vi "Agilis-Commands.vi"(6 "raw in":string="1ve?\r\n", 7 "Command in":T1(ring), 8 "error in (no error)":errorcluster, 9 "Value":dbl, 10 "Axis in":u8=1, 11 "VISA Refnum in":refnum<visa-resource-name>) -> (0 "error out":errorcluster, 1 "value":dbl format="%#.6g", 3 "VISA resource name out":refnum<visa-resource-name>, 4 "read buffer":string)   [LabVIEW 2011]
uses:
  <vilib>/Instr/_visa.llb/VISA Flush IO Buffer Mask.ctl
panel:
  out "sent":string
  out "return count":u32
  # "Staus x28: moving\nstatus x33_d51: OK\nstatus 10: no init?\nError 64:OK\nError:72 no init"
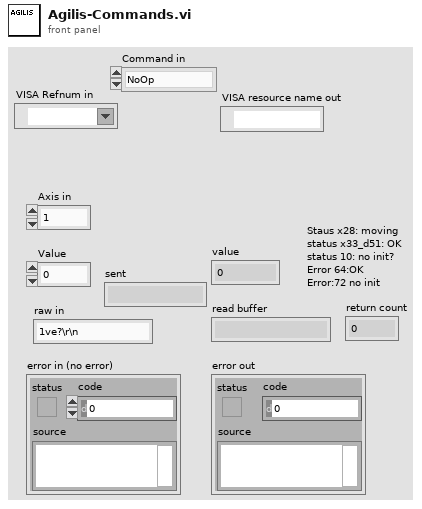
[diagram p1: front panel]
types:
  T1 = enum16{"NoOp", "GetStatus", "GetPosition", "SetPosition", "SetRelative", "GetError", "WriteRawAndRead", "clear", "switchOn"}
  T2 = typedef "VISA Flush IO Buffer Mask.ctl" = u16
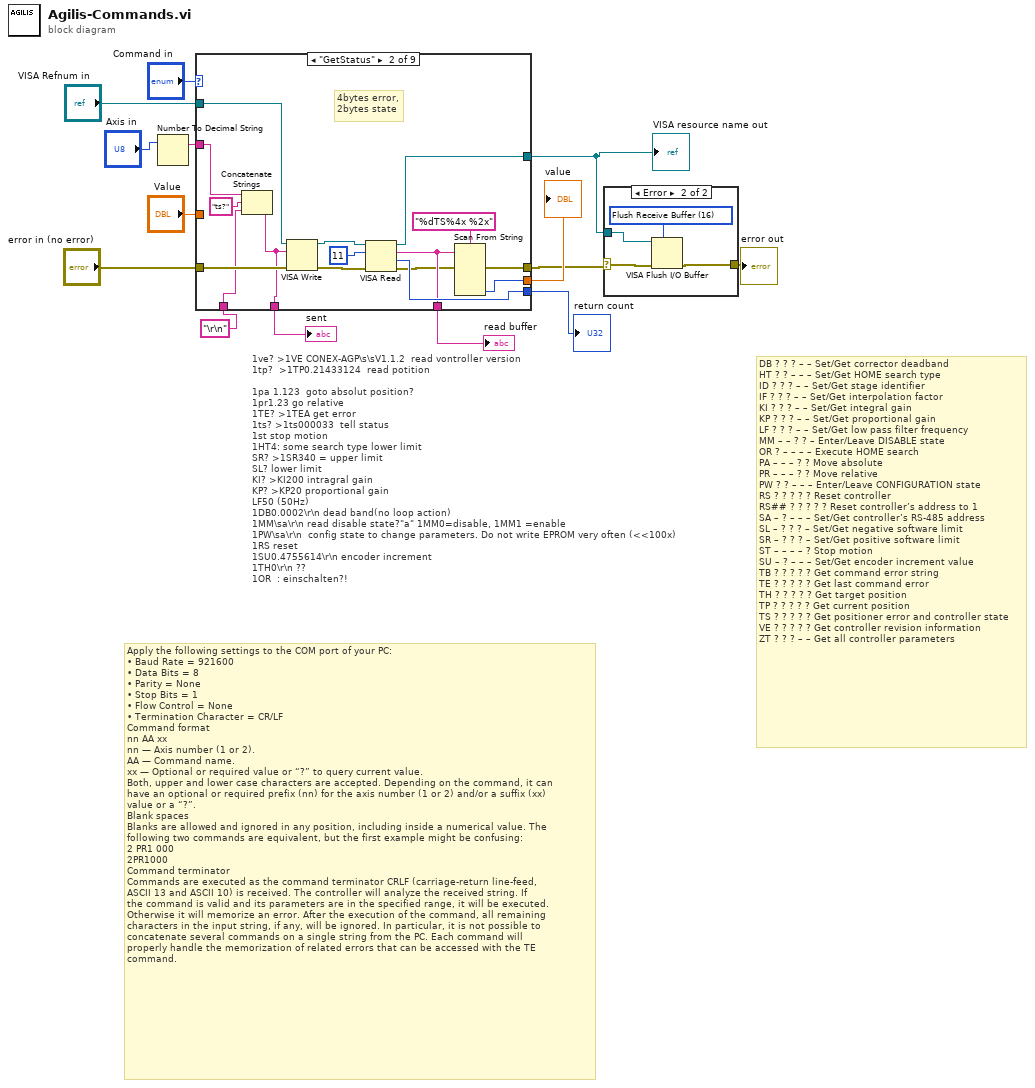
[diagram p0: block diagram]
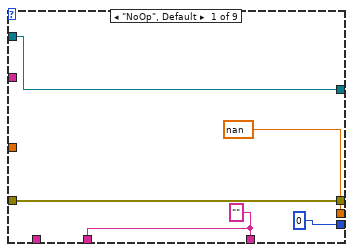
[diagram p3: hidden frame]
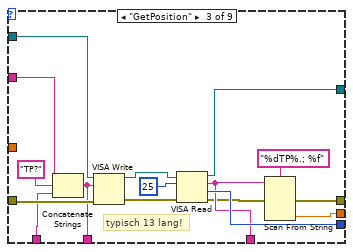
[diagram p4: hidden frame]
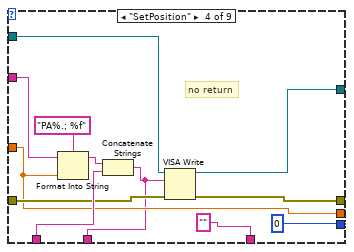
[diagram p5: hidden frame]
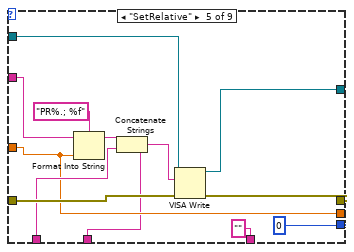
[diagram p6: hidden frame]
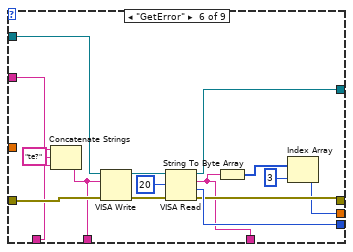
[diagram p7: hidden frame]
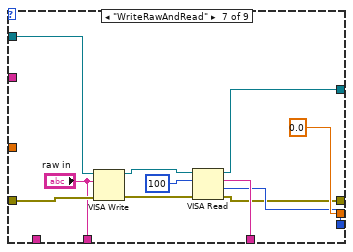
[diagram p8: hidden frame]
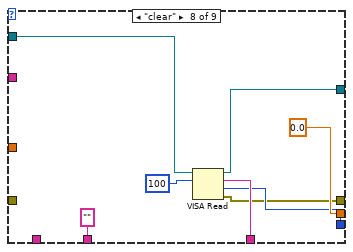
[diagram p9: hidden frame]
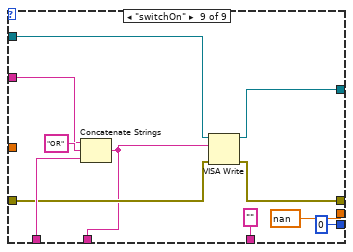
[diagram p10: hidden frame]
diagram:
  # "DB ? ? ? – – Set/Get corrector deadband \nHT ? ? – – – Set/Get HOME search type \nID ? ? ? – – Set/Get stage identifier \nIF ? ? ? – – Set/Get interpolation factor \nKI ? ? ? – – Set/Get integral gain \nKP ? ? ? – – Set/Get proportional gain \nLF ? ? ? – – Set/Get low pass filter frequency\nMM – – ? ? – Enter/Leave DISABLE state \nOR ? – – – – Execute HOME search \nPA – – – ? ? Move absolute \nPR – – – ? ? Move relative \nPW ? ? – – – Enter/Leave CONFIGURATION state \nRS ? ? ? ? ? Reset controller \nRS## ? ? ? ? ? Reset controller’s address to 1 \nSA – ? – – – Set/Get controller’s RS-485 address \nSL – ? ? ? – Set/Get negative software limit \nSR – ? ? ? – Set/Get positive software limit \nST – – – – ? Stop motion \nSU – ? – – – Set/Get encoder increment value \nTB ? ? ? ? ? Get command error string \nTE ? ? ? ? ? Get last command error \nTH ? ? ? ? ? Get target position \nTP ? ? ? ? ? Get current position \nTS ? ? ? ? ? Get positioner error and controller state \nVE ? ? ? ? ? Get controller revision information \nZT ? ? ? – – Get all controller parameters"
  # "Apply the following settings to the COM port of your PC:\n• Baud Rate = 921600\n• Data Bits = 8\n• Parity = None\n• Stop Bits = 1\n• Flow Control = None\n• Termination Character = CR/LF\nCommand format\nnn AA xx\nnn — Axis number (1 or 2).\nAA — Command name.\nxx — Optional or required value or “?” to query current value.\nBoth, upper and lower case characters are accepted. Depending on the command, it can \nhave an optional or required prefix (nn) for the axis number (1 or 2) and/or a suffix (xx) \nvalue or a “?”.\nBlank spaces\nBlanks are allowed and ignored in any position, including inside a numerical value. The \nfollowing two commands are equivalent, but the first example might be confusing:\n2 PR1 000\n2PR1000\nCommand terminator\nCommands are executed as the command terminator CRLF (carriage-return line-feed, \nASCII 13 and ASCII 10) is received. The controller will analyze the received string. If \nthe command is valid and its parameters are in the specified range, it will be executed. \nOtherwise it will memorize an error. After the execution of the command, all remaining \ncharacters in the input string, if any, will be ignored. In particular, it is not possible to \nconcatenate several commands on a single string from the PC. Each command will \nproperly handle the memorization of related errors that can be accessed with the TE \ncommand."
  # "1ve? >1VE CONEX-AGP\\s\\sV1.1.2  read vontroller version\n1tp?  >1TP0.21433124  read potition\n\n1pa 1.123  goto absolut position?\n1pr1.23 go relative\n1TE? >1TEA get error\n1ts? >1ts000033  tell status\n1st stop motion\n1HT4: some search type lower limit\nSR? >1SR340 = upper limit\nSL? lower limit\nKI? >KI200 intragral gain\nKP? >KP20 proportional gain\nLF50 (50Hz)\n1DB0.0002\\r\\n dead band(no loop action)\n1MM\\sa\\r\\n read disable state?\"a\" 1MM0=disable, 1MM1 =enable  \n1PW\\sa\\r\\n  config state to change parameters. Do not write EPROM very often (<<100x)\n1RS reset\n1SU0.4755614\\r\\n encoder increment\n1TH0\\r\\n ??\n1OR  : einschalten?!"
  n1 = Number To Decimal String(number="Axis in") -> (decimal integer string=w6:string)  [unwired: 1 in]
  n2 = case shown="\"GetStatus\"" "Command in" {
    tunnel: "Value" -> [_ _ _ w58 w66 _ _ _ _]
    tunnel: w6 -> [_ w26 w39 w53 w65 w79 _ _ w120]
    tunnel: [nan w20 w42 w58 w66 w82 0.0 0.0 nan ("Value")] -> w13
    tunnel: [w19 w22 w37 w55 w69 w84 w92 w105 w115] -> w3
    tunnel: "error in (no error)" -> [w19 w31 w46 w59 w72 w87 w98 _ w116]
    tunnel: "VISA Refnum in" -> [w18 w30 w47 w60 w73 w88 w99 w104 w118]
    tunnel: [w18 w29 w45 w57 w70 w86 w93 w106 w117] -> w1
    tunnel: [u32 0 ("return count") w28 w44 u32 0 ("byte count") u32 0 ("return count") w85 w95 w107 u32 0 ("return count")] -> w10
    tunnel: [w15 w27 w41 "" ("read buffer") "" ("read buffer") w81 w97 w109 "" ("read buffer")] -> w8
    tunnel: "\r\n" ("write buffer") -> [_ w24 w43 w61 w71 w77 _ _ w119]
    tunnel: [w15 w21 w36 w52 w64 w76 "raw in" "" ("raw in") w114] -> w4
    frame "NoOp", Default {
      w15 = "" ("read buffer")
    }
    frame "GetStatus" {
      # "4bytes error,\n2bytes state"
      n3 = Concatenate Strings(w26, "ts?" ("write buffer"), w24) -> (w21:string)
      n4 = VISA Write(VISA resource name=w30, write buffer=w21, error in (no error)=w31) -> (VISA resource name out=w32:refnum<visa-resource-name>, error out=w33:errorcluster)  [unwired: 1 out]
      n5 = VISA Read(VISA resource name=w32, byte count=u32 11, error in (no error)=w33) -> (VISA resource name out=w29:refnum<visa-resource-name>, read buffer=w27:string, return count=w28:u32, error out=w23:errorcluster)
      n6 = Scan From String(format string="%dTS%4x %2x", input string=w27, error in=w23) -> (error out=w22:errorcluster, output 3=w20:i32)  [unwired: 6 in, 2 out]
    }
    frame "GetPosition" {
      # "typisch 13 lang!"
      n7 = Concatenate Strings(w39, "TP?" ("format string"), w43) -> (w36:string)
      n8 = VISA Write(VISA resource name=w47, write buffer=w36, error in (no error)=w46) -> (VISA resource name out=w48:refnum<visa-resource-name>, error out=w49:errorcluster)  [unwired: 1 out]
      n9 = VISA Read(VISA resource name=w48, byte count=u32 25, error in (no error)=w49) -> (VISA resource name out=w45:refnum<visa-resource-name>, read buffer=w41:string, return count=w44:u32, error out=w38:errorcluster)
      n10 = Scan From String(format string="%dTP%.; %f", input string=w41, error in=w38) -> (error out=w37:errorcluster, output 2=w42:dbl)  [unwired: 4 in, 2 out]
    }
    frame "SetPosition" {
      # "no return"
      n11 = Format Into String(format string="PA%.; %f", initial string=w53, w58) -> (resulting string=w62:string)  [unwired: 1 in, 1 out]
      n12 = Concatenate Strings(w62, w61) -> (w52:string)
      n13 = VISA Write(VISA resource name=w60, write buffer=w52, error in (no error)=w59) -> (VISA resource name out=w57:refnum<visa-resource-name>, error out=w55:errorcluster)  [unwired: 1 out]
    }
    frame "SetRelative" {
      n14 = Format Into String(format string="PR%.; %f", initial string=w65, w66) -> (resulting string=w74:string)  [unwired: 1 in, 1 out]
      n15 = Concatenate Strings(w74, w71) -> (w64:string)
      n16 = VISA Write(VISA resource name=w73, write buffer=w64, error in (no error)=w72) -> (VISA resource name out=w70:refnum<visa-resource-name>, error out=w69:errorcluster)  [unwired: 1 out]
    }
    frame "GetError" {
      n17 = Concatenate Strings(w79, "te?" ("write buffer"), w77) -> (w76:string)
      n18 = VISA Write(VISA resource name=w88, write buffer=w76, error in (no error)=w87) -> (VISA resource name out=w89:refnum<visa-resource-name>, error out=w90:errorcluster)  [unwired: 1 out]
      n19 = VISA Read(VISA resource name=w89, byte count=u32 20, error in (no error)=w90) -> (VISA resource name out=w86:refnum<visa-resource-name>, read buffer=w81:string, return count=w85:u32, error out=w84:errorcluster)
      n20 = String To Byte Array(string=w81) -> (unsigned byte array=w83:u8[])
      n21 = Index Array(array=w83, index=3) -> (element=w82:u8)
    }
    frame "WriteRawAndRead" {
      n22 = VISA Write(VISA resource name=w99, write buffer="raw in", error in (no error)=w98) -> (VISA resource name out=w100:refnum<visa-resource-name>, error out=w101:errorcluster)  [unwired: 1 out]
      n23 = VISA Read(VISA resource name=w100, byte count=u32 100, error in (no error)=w101) -> (VISA resource name out=w93:refnum<visa-resource-name>, read buffer=w97:string, return count=w95:u32, error out=w92:errorcluster)
    }
    frame "clear" {
      n24 = VISA Read(VISA resource name=w104, byte count=u32 100) -> (VISA resource name out=w106:refnum<visa-resource-name>, read buffer=w109:string, return count=w107:u32, error out=w105:errorcluster)  [unwired: 1 in]
    }
    frame "switchOn" {
      n25 = Concatenate Strings(w120, "OR", w119) -> (w114:string)
      n26 = VISA Write(VISA resource name=w118, write buffer=w114, error in (no error)=w116) -> (VISA resource name out=w117:refnum<visa-resource-name>, error out=w115:errorcluster)  [unwired: 1 out]
    }
  }
  "value" <- w13
  "VISA resource name out" <- w1
  "return count" <- w10
  "read buffer" <- w8
  "sent" <- w4
  n27 = case shown="Error" w3 {
    selector: w3 -> [w122 w125]
    tunnel: [w122 w124] -> w2
    tunnel: w1 -> [_ w126]
    frame No Error {
    }
    frame Error {
      w123 = T2 16 items=["Flush Receive Buffer"=16, "Write Transmit Buffer to Device"=32, "Flush Receive Buffer (No I/O)"=64, "Flush Transmit Buffer"=128] ("Mask")
      n28 = VISA Flush I/O Buffer(VISA resource name=w126, mask (16)=w123, error in (no error)=w125) -> (error out=w124:errorcluster)  [unwired: 1 out]
    }
  }
  "error out" <- w2
